vi "Refresh User.vi"(8 "error in (no error)":errorcluster, 10 "User In":refnum<class "User.lvclass">, 11 "User DB in":refnum<class "User DB.lvclass">) -> (0 "error out":errorcluster, 2 "User":refnum<class "User.lvclass">, 3 "User DB out":refnum<class "User DB.lvclass">)   [LabVIEW 2020, in "Summer of LabVIEW.lvlib" / "User DB.lvclass"]
uses:
  User DB.lvclass
  <vilib>/IlluminatedG/IG HTTP Server/HTTP Server/User/User.lvclass
  User DB.lvclass/User DB.ctl
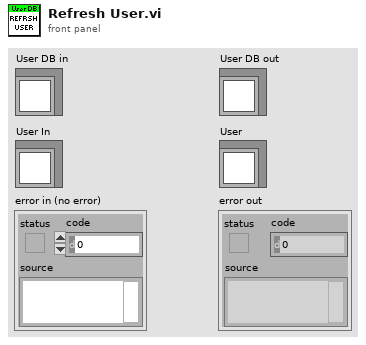
[diagram p1: front panel]
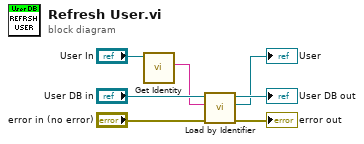
[diagram p0: block diagram]
diagram:
  n1 = call-dynamic "Get Identity.vi"("User in"="User In") -> ("Identity"=w1:string)  [unwired: 8 in, 2 out]
  n2 = call-dynamic "Load by Identifier.vi"("error in (no error)"="error in (no error)", "Identifier"=w1, "User DB in"="User DB in") -> ("error out"=→"error out":errorcluster, "User"=→"User":refnum<class "User.lvclass">, "User DB out"=→"User DB out":refnum<class "User DB.lvclass">)  [unwired: 6 in]
